vi "vi-icon.get.vi"(8 "error in":errorcluster, 11 "VI in":refnum<vi>) -> (0 "error out":errorcluster, 2 "VI Icon":picture, 3 "VI out":refnum<vi>)   [LabVIEW 2020]
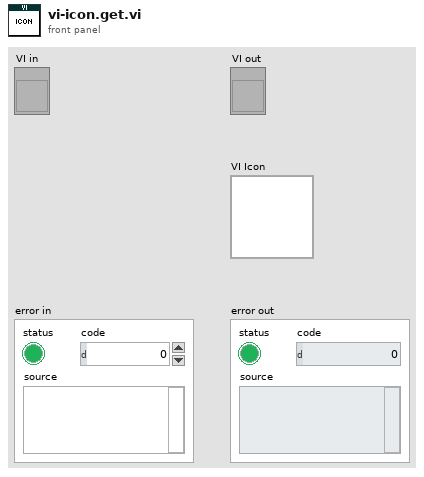
[diagram p1: front panel]
types:
  T1 = typedef "imagedata.ctl" = cluster{"image type":i32, "image depth":i32, "image":u8[], "mask":u8[], "colors":u32[], "Rectangle":cluster{"left":i16, "top":i16, "right":i16, "bottom":i16}}
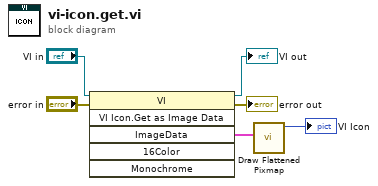
[diagram p0: block diagram]
diagram:
  n1 = invoke class="VI" method="VI Icon.Get as Image Data"(reference="VI in", error in="error in") -> (reference out=→"VI out":refnum<vi>, error out=→"error out":errorcluster, "ImageData"=w5:T1)  [unwired: 4 in, 3 out]
  n2 = call <vilib>:"Draw Flattened Pixmap.vi"("image data"=w5) -> ("new picture"=→"VI Icon":picture)  [unwired: 8 in]
